vi "configure shutdown action UI.vi"(8 "error in (no error)":errorcluster, 9 "supported actions list":T1[](array[typedef]), 10 "user event":refnum<user-event>, 11 "Simple Sequencer TBM configuration":refnum<class "Simple Sequencer TBM configuration.lvclass">) -> (0 "error out":errorcluster, 3 "Simple Sequencer TBM configuration":refnum<class "Simple Sequencer TBM configuration.lvclass">)   [LabVIEW 2014, in "Simple Sequencer TBM editor node.lvclass"]
doc: "Dialog allowing users to configure what action to run in safe state."
uses:
  Simple Sequencer TBM editor node.lvclass
  module/configuration/Simple Sequencer TBM configuration.lvclass
  user event typedef.ctl
  action config and UI pairing.ctl
  sequencer parent classes/action configuration parent/action configuration.lvclass
  subpanel state.ctl
  VI calling template typedef.ctl
  module/configuration/Simple Sequencer TBM configuration.lvclass/Simple Sequencer TBM configuration.ctl
  module/configuration/Write shutdown action config.vi
  module/configuration/Read shutdown action config.vi
panel:
  in  "Remove":bool
  in  "Cancel":bool
  in  "Save":bool
  in  "Select Action":bool
  out "Shutdown Action":string
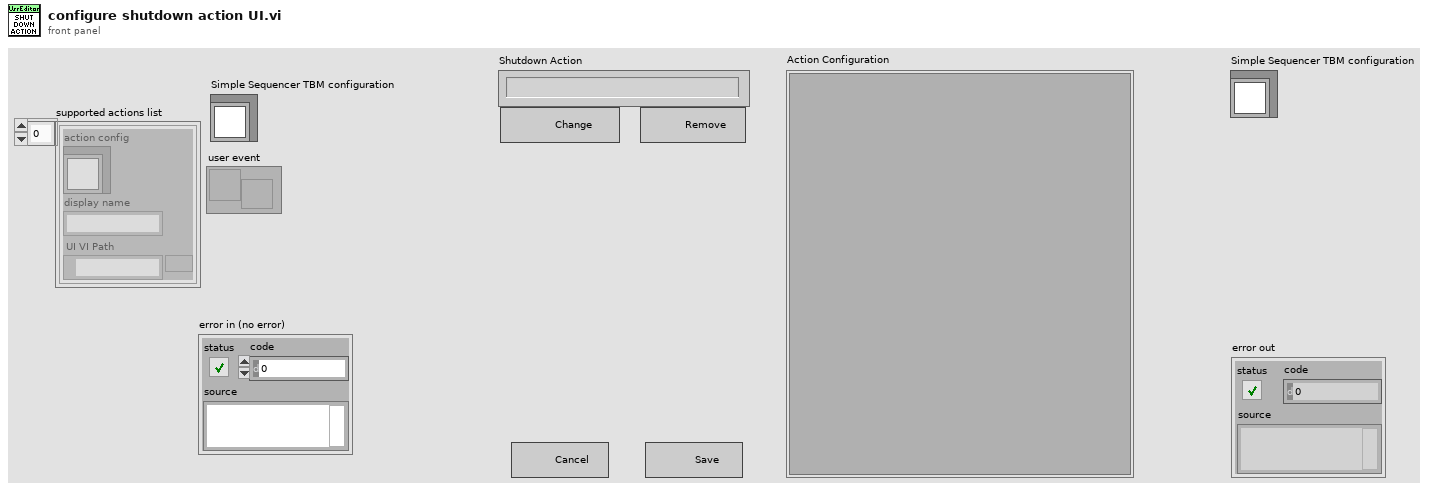
[diagram p1: front panel]
types:
  T1 = typedef "Simple Sequencer TBM editor node.lvclass/action config and UI pairing.ctl" = cluster{"action config":refnum<class "action configuration.lvclass">, "display name":string, "UI VI Path":path}
  T2 = typedef "Simple Sequencer TBM editor node.lvclass/subpanel state.ctl" = cluster{"active VI":T3, "action UI user event":refnum<user-event>, "SubPnl Refnum":refnum<vi>, "supported actions list":T1[]}
  T3 = typedef "Simple Sequencer TBM editor node.lvclass/VI calling template typedef.ctl" = refnum<vi>
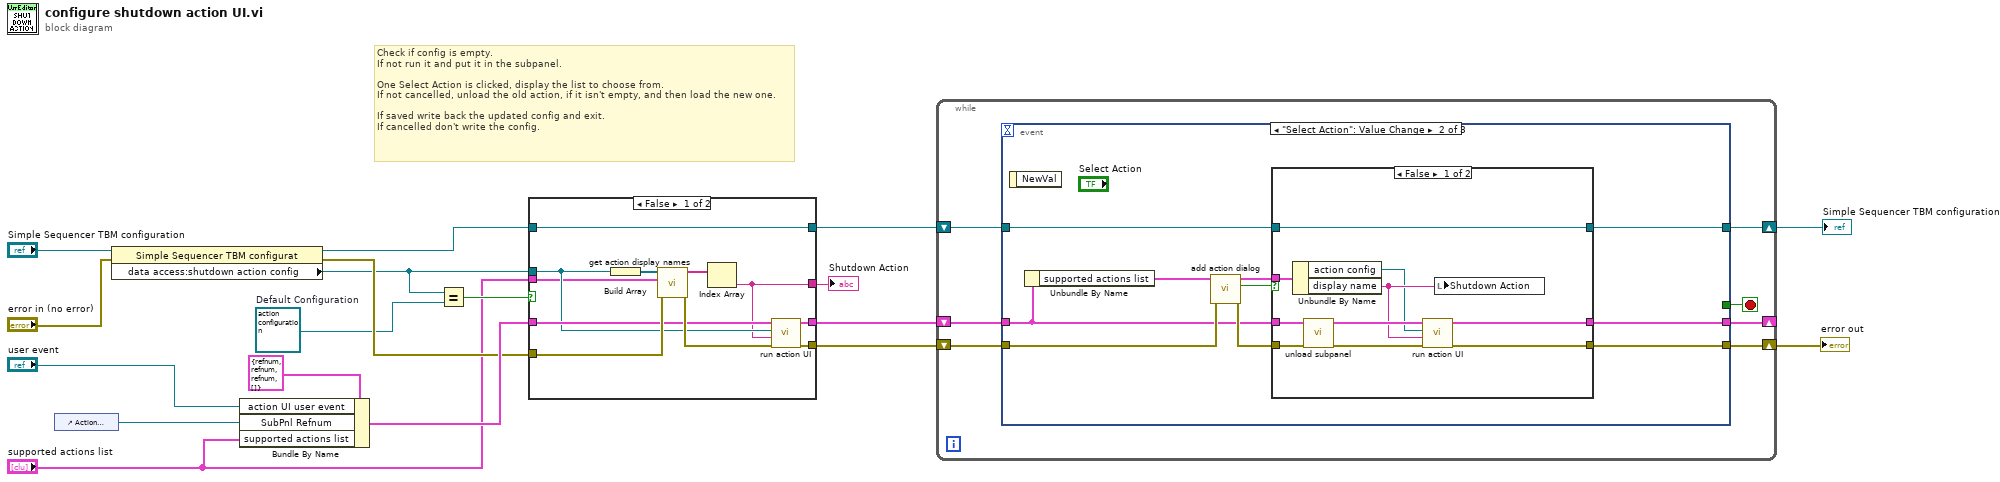
[diagram p0: block diagram]
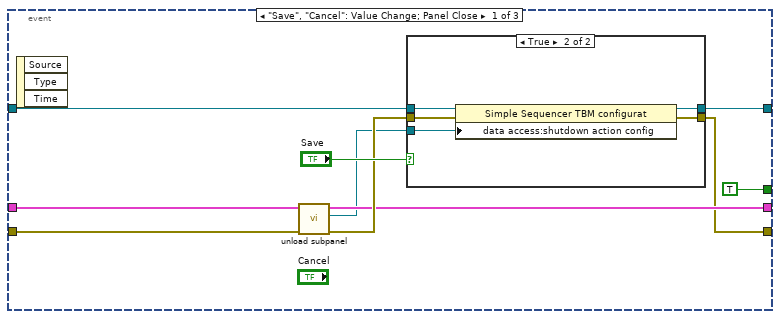
[diagram p3: hidden frame]
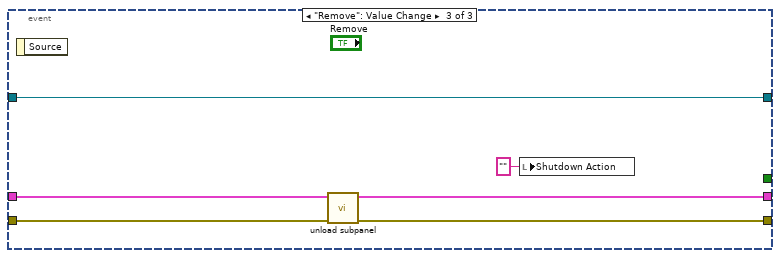
[diagram p6: hidden frame]
diagram:
  w5 = refnum<class "action configuration.lvclass"> refnum  # Default Configuration
  # "Check if config is empty.\nIf not run it and put it in the subpanel.\n\nOne Select Action is clicked, display the list to choose from.\nIf not cancelled, unload the old action, if it isn't empty, and then load the new one.\n\nIf saved write back the updated config and exit.\nIf cancelled don't write the config."
  n1 = control-ref of="Action Configuration"() -> (w11:refnum<vi>)
  n2 = property class="Simple Sequencer TBM configurat"(reference="Simple Sequencer TBM configuration", error in="error in (no error)") -> (reference out=w14:refnum<class "Simple Sequencer TBM configuration.lvclass">, error out=w6:errorcluster, "data access:shutdown action config"=w3:refnum<class "action configuration.lvclass">)
  n3 = Bundle By Name(cluster=T2 {"active VI"=refnum, "action UI user event"=refnum, "SubPnl Refnum"=refnum, "supported actions list"=[]} ("subpanel state"), "action UI user event"="user event", "SubPnl Refnum"=w11, "supported actions list"="supported actions list") -> (w9:T2)
  n4 = Equal?(x=w3, y=w5) -> (x = y?=w4:bool)
  n5 = case shown="False" w4 {
    tunnel: [w23 w30] -> w16
    tunnel: [w22 w32] -> w15
    tunnel: w3 -> [w21 _]
    tunnel: w6 -> [w26 w32]
    tunnel: w14 -> [w25 w31]
    tunnel: [w25 w31] -> w13
    tunnel: w9 -> [w24 w30]
    tunnel: [w20 _] -> w2
    tunnel: "supported actions list" -> [w19 _]
    frame False {
      n6 = Build Array(w21) -> (w29:refnum<class "action configuration.lvclass">[])
      n7 = call "get action display names.vi"("error in (no error)"=w26, "supported actions list"=w19, "action configs"=w29) -> ("error out"=w27:errorcluster, "display names"=w28:string[])  [unwired: 7 in]
      n8 = Index Array(array=w28) -> (element=w20:string)  [unwired: 1 in]
      n9 = call "run action UI.vi"("error in (no error)"=w27, "action display name"=w20, "action configuration"=w21, "subpanel state"=w24) -> ("error out"=w22:errorcluster, "subpanel state out"=w23:T2)  [unwired: 6 in]
    }
    frame True {
    }
  }
  "Shutdown Action" <- w2
  n10 = while {
    shift-right: [w33] -> w7
    shift-left: w13 -> [w34]
    shift-right: [w35] -> w8
    shift-left: w15 -> [w36]
    shift-right: [w37] -> _
    shift-left: w16 -> [w38]
    stop <- w39 stop-if-true
    n11 = event shown="[1] \"Select Action\": Value Change" {
      selector: _ -> [_ _ _]
      dyn-events: _ -> [_ _ _]
      timeout: _ -> [_ _ _]
      tunnel: [TRUE _ _] -> w39
      tunnel: w38 -> [w48 w58 w84]
      tunnel: [w42 w66 w82] -> w37
      tunnel: w36 -> [w47 w64 w83]
      tunnel: [w41 w65 w81] -> w35
      tunnel: w34 -> [w45 w60 w85]
      tunnel: [w43 w59 w85] -> w33
      event "Save", "Cancel": Value Change; Panel Close {
        n12 = event-data() -> ()  [unwired: 1 in, 3 out]
        n13 = call "unload subpanel.vi"("error in (no error)"=w47, "subpanel state"=w48) -> ("error out"=w44:errorcluster, "action configuration out"=w40:refnum<class "action configuration.lvclass">, "subpanel state out"=w42:T2)  [unwired: 6 in, 1 out]
        n14 = case shown="True" "Save" {
          tunnel: w45 -> [w51 w56]
          tunnel: w44 -> [w50 w55]
          tunnel: [w51 w54] -> w43
          tunnel: [w50 w53] -> w41
          tunnel: w40 -> [_ w52]
          frame False {
          }
          frame True {
            n15 = property class="Simple Sequencer TBM configurat"(reference=w56, error in=w55, "data access:shutdown action config"=w52) -> (reference out=w54:refnum<class "Simple Sequencer TBM configuration.lvclass">, error out=w53:errorcluster)
          }
        }
      }
      event "Select Action": Value Change {
        n16 = event-data() -> ()  [unwired: 1 in, 1 out]
        n17 = Unbundle By Name(w58) -> ("supported actions list"=w57:T1[])
        n18 = call "add action dialog.vi"("error in (no error)"=w64, "supported actions list"=w57) -> ("error out"=w63:errorcluster, "cancelled"=w62:bool, "config and UI pairing"=w61:T1)  [unwired: 7 in]
        n19 = case shown="False" w62 {
          tunnel: w58 -> [w76 w78]
          tunnel: [w72 w78] -> w66
          tunnel: [w71 w77] -> w65
          tunnel: w63 -> [w75 w77]
          tunnel: w61 -> [w74 _]
          tunnel: w60 -> [w69 w79]
          tunnel: [w69 w79] -> w59
          frame False {
            n20 = Unbundle By Name(w74) -> ("action config"=w67:refnum<class "action configuration.lvclass">, "display name"=w68:string)
            n21 = call "unload subpanel.vi"("error in (no error)"=w75, "subpanel state"=w76) -> ("error out"=w70:errorcluster, "subpanel state out"=w73:T2)  [unwired: 6 in, 2 out]
            n22 = call "run action UI.vi"("error in (no error)"=w70, "action display name"=w68, "action configuration"=w67, "subpanel state"=w73) -> ("error out"=w71:errorcluster, "subpanel state out"=w72:T2)  [unwired: 6 in]
            n23 = local write "Shutdown Action"(w68) -> ()
          }
          frame True {
          }
        }
      }
      event "Remove": Value Change {
        n24 = event-data() -> ()  [unwired: 1 in, 1 out]
        n25 = call "unload subpanel.vi"("error in (no error)"=w83, "subpanel state"=w84) -> ("error out"=w81:errorcluster, "subpanel state out"=w82:T2)  [unwired: 6 in, 2 out]
        n26 = local write "Shutdown Action"("" ("Shutdown Action")) -> ()
      }
    }
  }
  "error out" <- w8
  "Simple Sequencer TBM configuration" <- w7
